vi "Compare Two Folders.vi"(8 "error in (no error)":errorcluster, 10 "appended path 2":path, 11 "appended path":path) -> (0 "error out":errorcluster, 1 "Contents are the same?":bool)   [LabVIEW 2019]
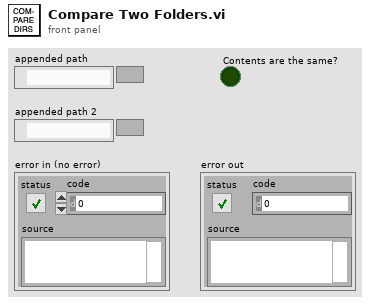
[diagram p1: front panel]
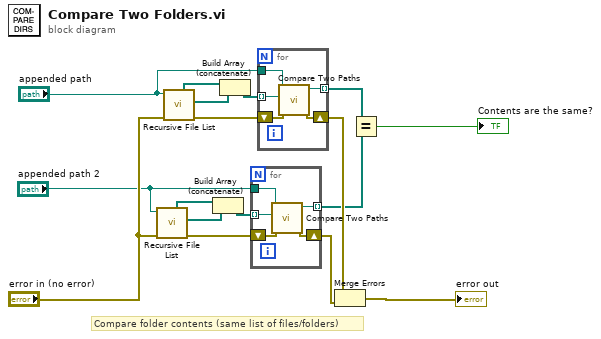
[diagram p0: block diagram]
diagram:
  # "Compare folder contents (same list of files/folders)"
  n1 = call <vilib>:"Recursive File List.vi"("error in (no error)"="error in (no error)", "Folder Path"="appended path 2") -> ("error out"=w7:errorcluster, "All Files in Dir"=w1:path[], "All Folders"=w3:path[])  [unwired: 5 in, 2 out]
  n2 = call <vilib>:"Recursive File List.vi"("error in (no error)"="error in (no error)", "Folder Path"="appended path") -> ("error out"=w8:errorcluster, "All Files in Dir"=w11:path[], "All Folders"=w10:path[])  [unwired: 5 in, 2 out]
  n3 = Build Array (concatenate)(w3, w1) -> (w4:path[])
  n4 = Build Array (concatenate)(w10, w11) -> (w9:path[])
  n5 = for {
    tunnel: w4 -> [w22] mode=indexing
    tunnel: "appended path 2" -> [w21]
    tunnel: [w20] -> w6 mode=indexing
    shift-right: [w18] -> w16
    shift-left: w7 -> [w19]
    n6 = call <vilib>:"Compare Two Paths.vi"("error in (no error)"=w19, "Path 2"=w22, "Path 1"=w21) -> ("error out"=w18:errorcluster, "Relative Path from 1 to 2"=w20:path)  [unwired: 5 in, 2 out]
  }
  n7 = for {
    tunnel: w9 -> [w27] mode=indexing
    tunnel: "appended path" -> [w26]
    tunnel: [w25] -> w14 mode=indexing
    shift-right: [w23] -> w15
    shift-left: w8 -> [w24]
    n8 = call <vilib>:"Compare Two Paths.vi"("error in (no error)"=w24, "Path 2"=w27, "Path 1"=w26) -> ("error out"=w23:errorcluster, "Relative Path from 1 to 2"=w25:path)  [unwired: 5 in, 2 out]
  }
  n9 = Merge Errors(w15, w16) -> (→"error out":errorcluster)
  n10 = Equal?(x=w14, y=w6) -> (x = y?=→"Contents are the same?":bool)
